vi "GetErrorCode.vi"(8 "error in (no error)":errorcluster) -> (0 "error out":errorcluster, 3 "Error Code":u32)   [LabVIEW 2014, in "LabBASSMOD2.lvlib"]
uses:
  LabBASSMOD2.lvlib
  DLL/BASSMOD.dll
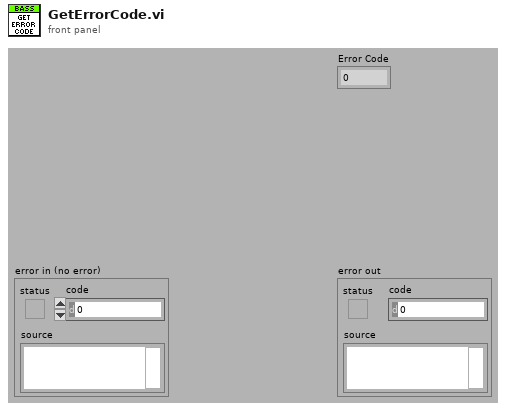
[diagram p1: front panel]
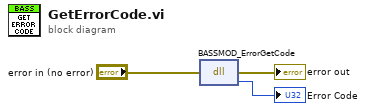
[diagram p0: block diagram]
diagram:
  n1 = dll-call lib="C:/dev/PGS/LabBASSMOD2/DLL/BASSMOD.dll" fn="BASSMOD_ErrorGetCode"(error in="error in (no error)") -> (error out=→"error out":errorcluster, "return type"=→"Error Code":u32)  [unwired: 2 in, 1 out]
